vi "LoadingWindow.vi"(11 "channel":T1) -> ()   [LabVIEW 2022 SP3]
uses:
  <extravilib>/ChannelInstances/Stream-str/)Channel.ctl
  <extravilib>/ChannelInstances/Tag-bool/Read With Abort.vi
  <extravilib>/ChannelInstances/Stream-str/Read With Abort.vi
  <extravilib>/ChannelInstances/Tag-bool/Write With Abort.vi
  <extravilib>/ChannelInstances/Stream-str/EndpointRead.vi
  <extravilib>/ChannelInstances/Tag-bool/Instantiate.vi
  <extravilib>/ChannelInstances/Tag-bool/EndpointRead.vi
  <extravilib>/ChannelInstances/Stream-str/)Channel.vi
  <resource>/ChannelSupport/_ChannelSupport/WaitIfNeeded.vi
  <extravilib>/ChannelInstances/Tag-bool/Endpoint.vi
  <extravilib>/ChannelInstances/Tag-bool.lvlib
  <extravilib>/ChannelInstances/Stream-str.lvlib
panel:
  out "DescriptionBuffer":string
  out "Progress":dbl(slide) scale=0.0..14.0
  out "Description":string
  out "Task":string
  out "Version":string
  # "Ice Nucleation Controller"
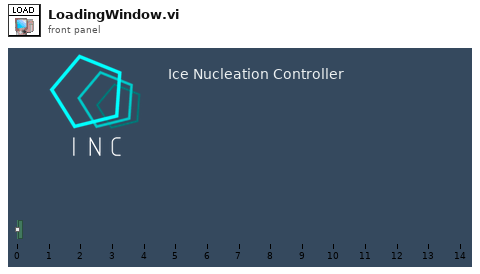
[diagram p1: front panel]
types:
  T1 = typedef "Stream-str.lvlib/)Channel.ctl" = refnum<queue>
  T2 = enum32{"Invalid", "Standard", "Closed", "Hidden", "Minimized", "Maximized"}
  T3 = enum32{"invalid app kind", "Development System", "Run Time System", "Student Edition", "Embedded LabVIEW", "Evaluation", "Custom"}
  T4 = cluster{"Core":cluster{"Current VI Reference":refnum<vi>, "Close Panel on Exit?":bool}, "Your Boolean data":bool, "Your string data":string}
  T5 = cluster{"Current VI Reference":refnum<vi>, "Close Panel on Exit?":bool}
  T6 = typedef "Tag-bool.lvlib/))Channel.ctl" = refnum<queue>
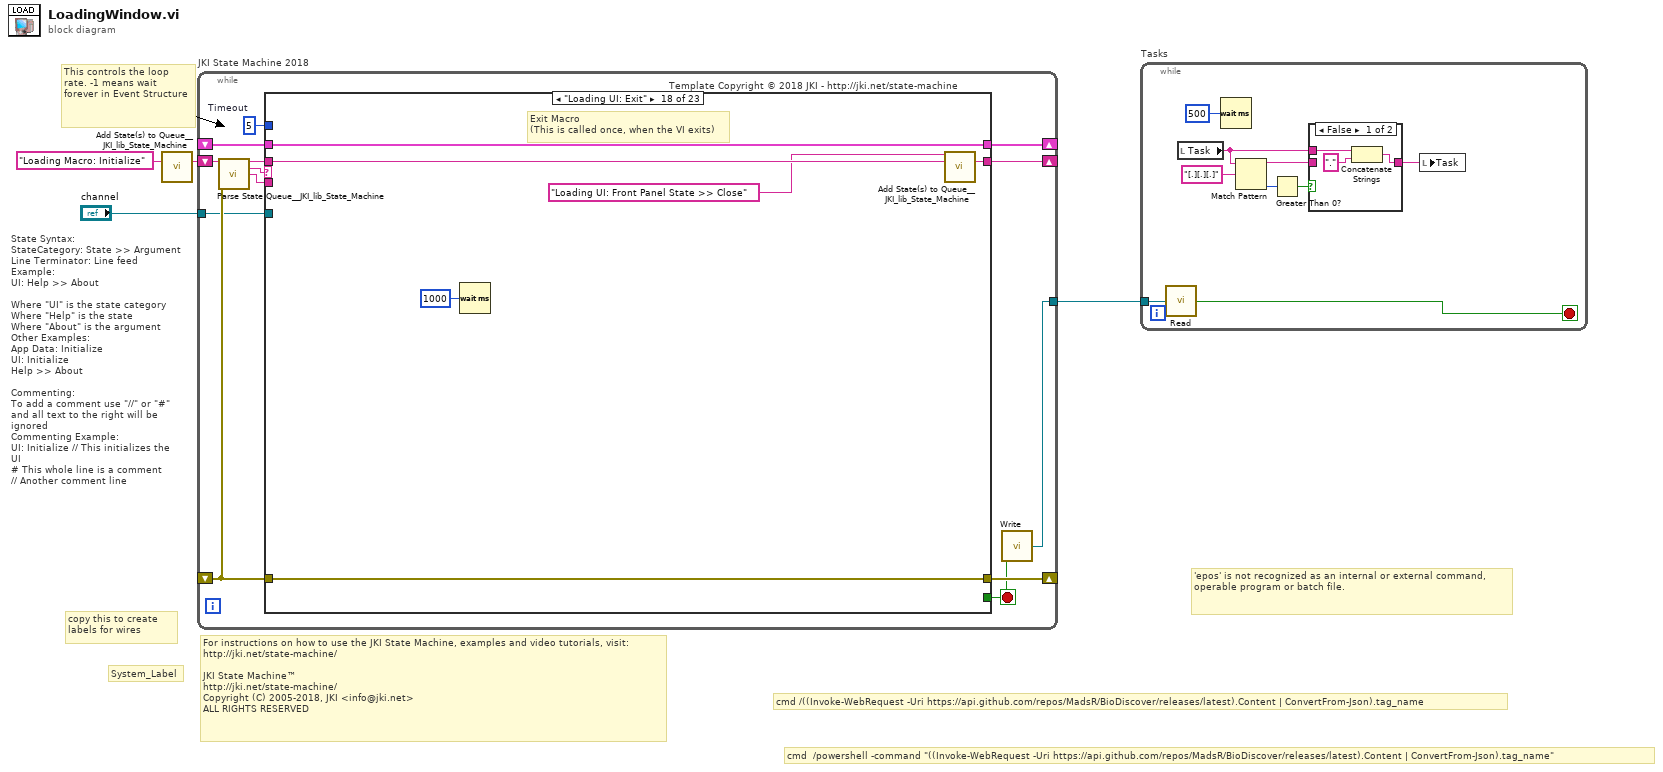
[diagram p0: block diagram]
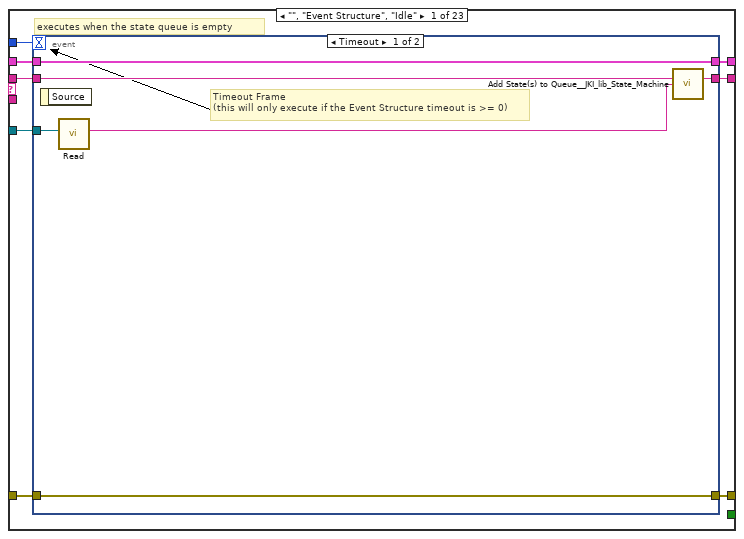
[diagram p3: hidden frame]
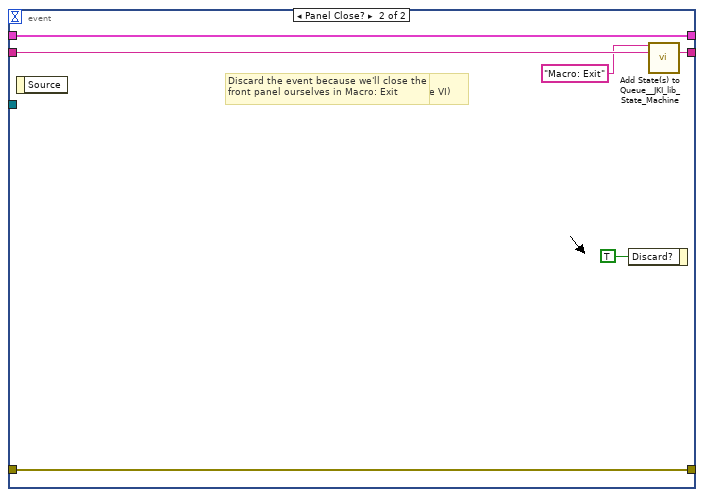
[diagram p4: hidden frame]
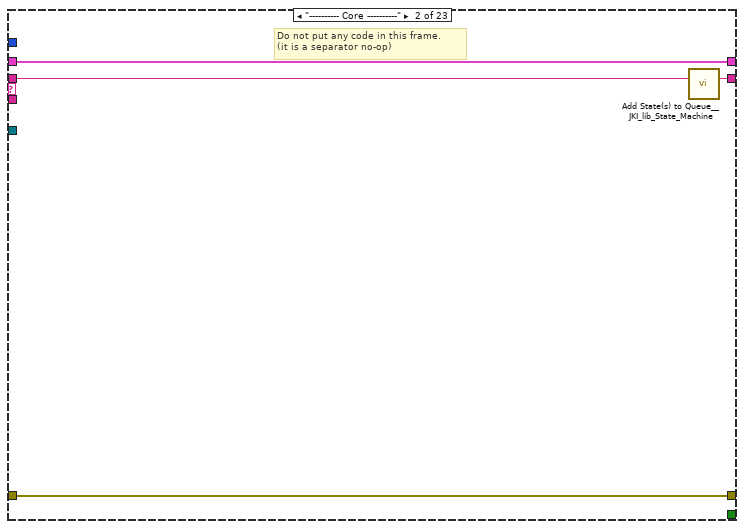
[diagram p5: hidden frame]
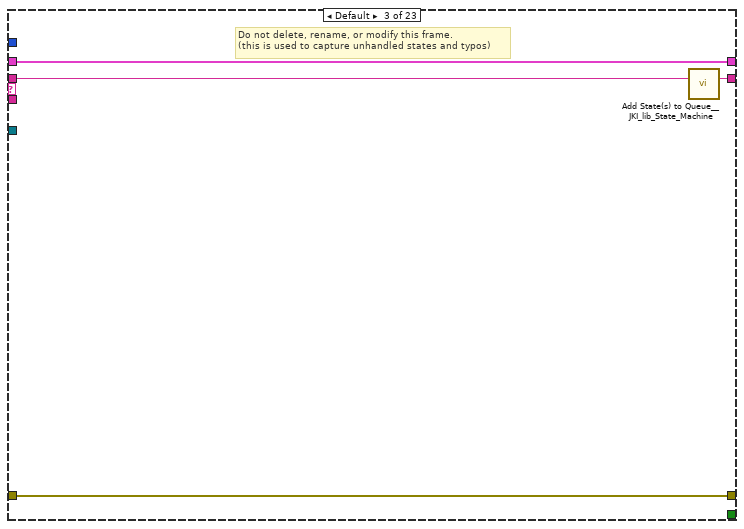
[diagram p6: hidden frame]
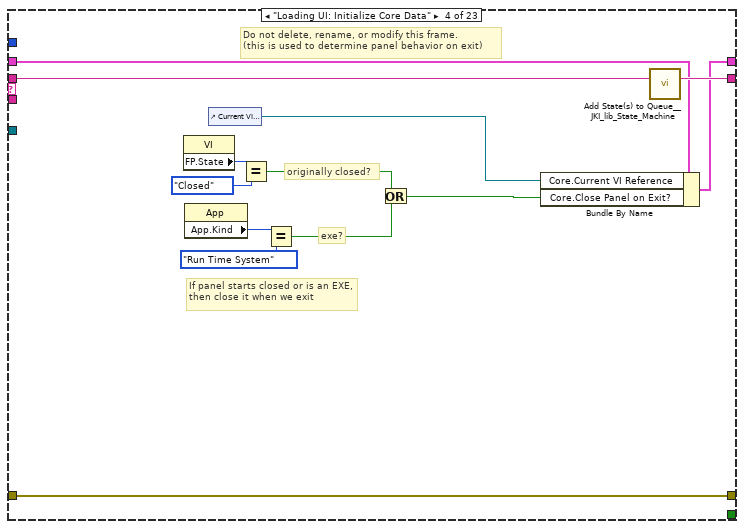
[diagram p7: hidden frame]
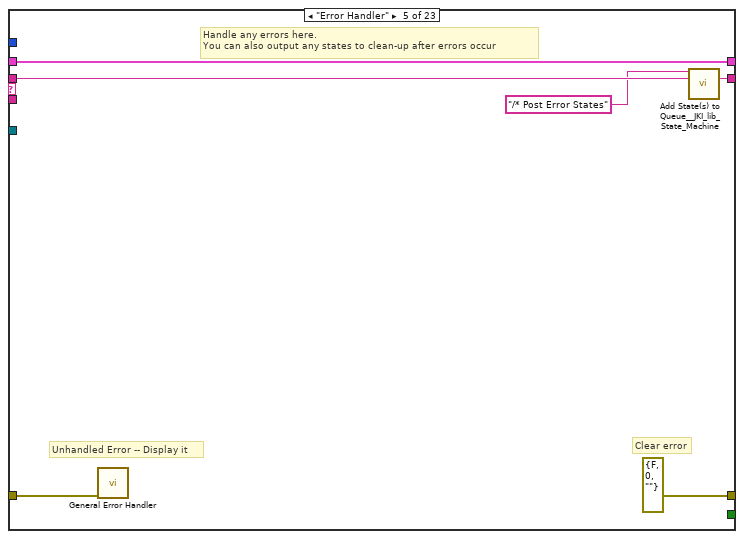
[diagram p8: hidden frame]
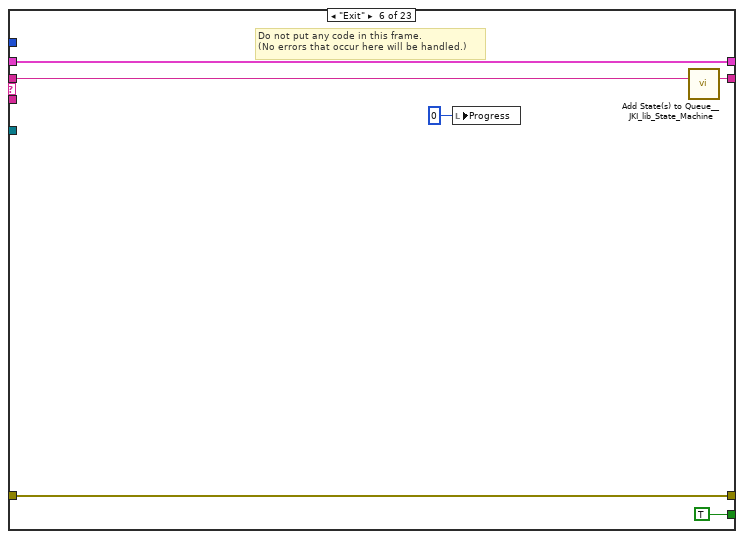
[diagram p9: hidden frame]
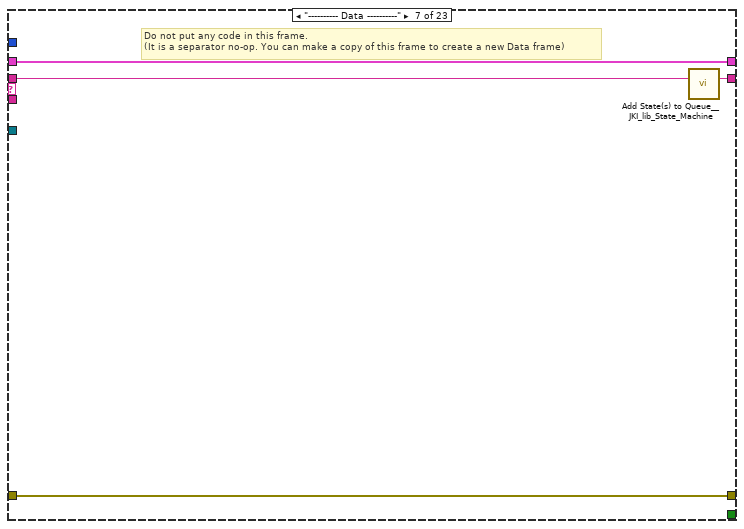
[diagram p10: hidden frame]
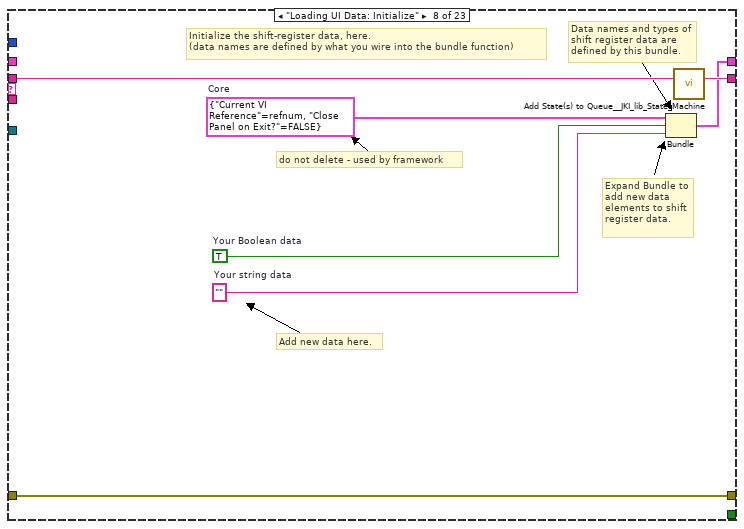
[diagram p11: hidden frame]
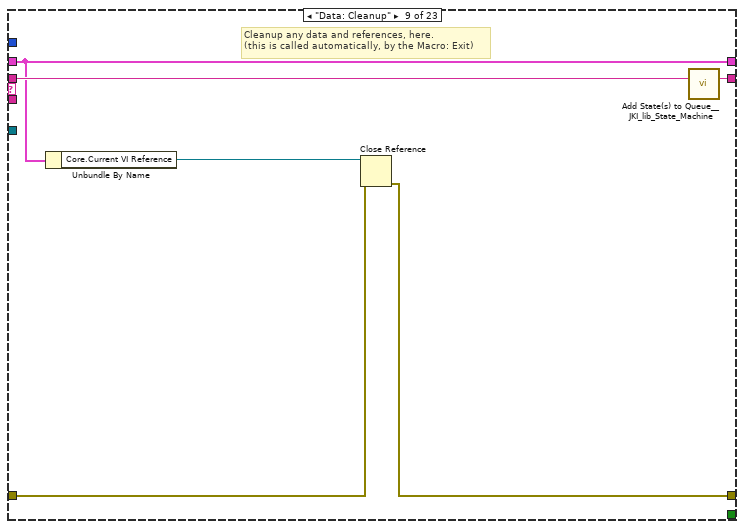
[diagram p12: hidden frame]
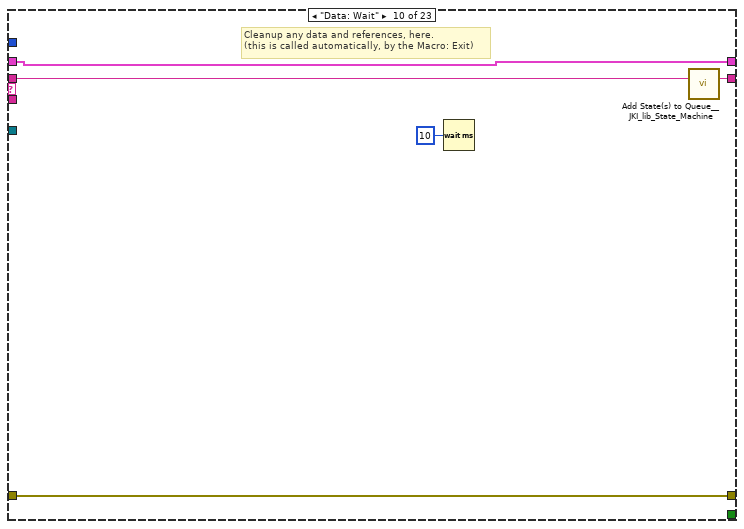
[diagram p13: hidden frame]
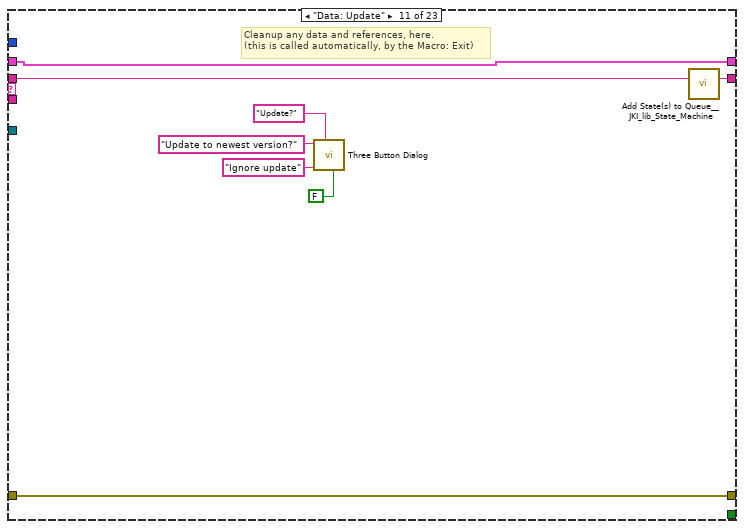
[diagram p14: hidden frame]
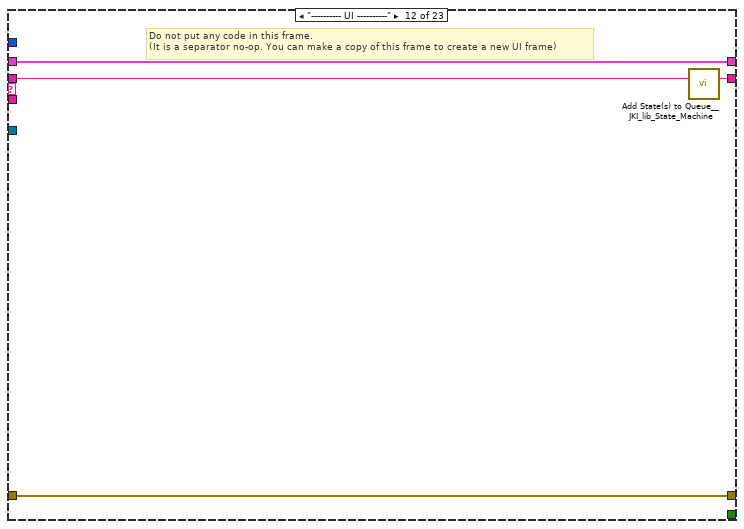
[diagram p15: hidden frame]
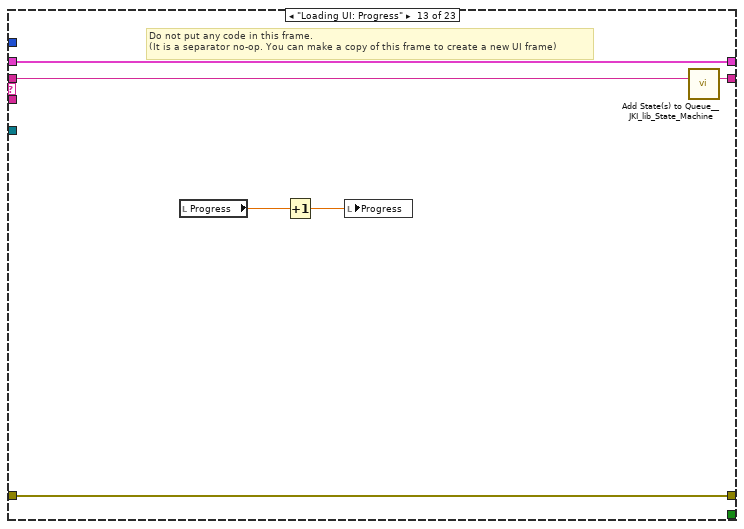
[diagram p16: hidden frame]
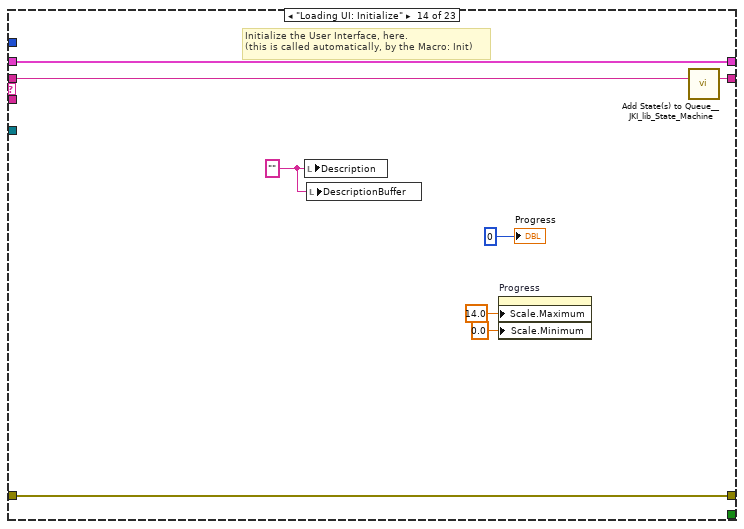
[diagram p17: hidden frame]
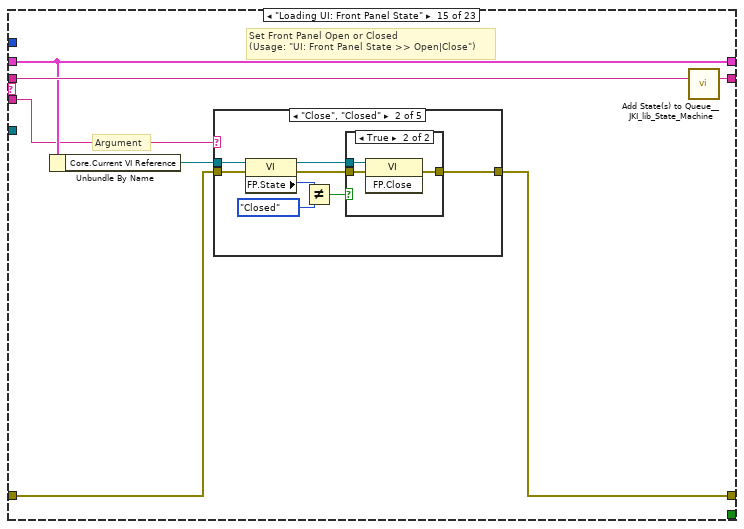
[diagram p18: hidden frame]
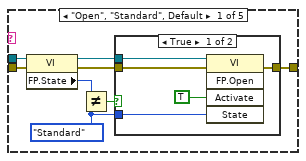
[diagram p19: hidden frame]
diagram:
  # "cmd  /powershell -command \"((Invoke-WebRequest -Uri https://api.github.com/repos/MadsR/BioDiscover/releases/latest).Content | ConvertFrom-Json).tag_name\""
  # "cmd /((Invoke-WebRequest -Uri https://api.github.com/repos/MadsR/BioDiscover/releases/latest).Content | ConvertFrom-Json).tag_name"
  # "'epos' is not recognized as an internal or external command,\noperable program or batch file."
  # "For instructions on how to use the JKI State Machine, examples and video tutorials, visit:\nhttp://jki.net/state-machine/\n\nJKI State Machine™\nhttp://jki.net/state-machine/\nCopyright (C) 2005-2018, JKI <info@jki.net>\nALL RIGHTS RESERVED"
  # "State Syntax:\nStateCategory: State >> Argument\nLine Terminator: Line feed\nExample:\nUI: Help >> About\n\nWhere \"UI\" is the state category\nWhere \"Help\" is the state\nWhere \"About\" is the argument\nOther Examples:\nApp Data: Initialize\nUI: Initialize\nHelp >> About\n\nCommenting:\nTo add a comment use \"//\" or \"#\" and all text to the right will be ignored\nCommenting Example:\nUI: Initialize // This initializes the UI\n# This whole line is a comment\n// Another comment line"
  # "copy this to create labels for wires"
  # "This controls the loop rate. -1 means wait forever in Event Structure"
  # "System_Label"
  n1 = call <vilib>:"Add State(s) to Queue__JKI_lib_State_Machine.vi"("State(s) in (\"\")"="Loading Macro: Initialize") -> ("States Out"=w4:string)  [unwired: 14 in]
  n2 = while "JKI State Machine 2018" {
    shift-right: [w10] -> _
    shift-left: _ -> [w9]
    shift-right: [w13] -> _
    shift-left: _ -> [w7]
    shift-right: [w12] -> _
    shift-left: w4 -> [w14]
    tunnel: [w6] -> w2
    tunnel: "channel" -> [w5]
    stop <- w11 stop-if-true
    w8 = 5  # Timeout
    # "Template Copyright © 2018 JKI - http://jki.net/state-machine"
    n3 = call <vilib>:"Parse State Queue__JKI_lib_State_Machine.vi"("State Queue"=w14, "Error In (no error)"=w7) -> ("Remaining States"=w16:string, "Current State"=w17:string, "Arguments"=w15:string)  [unwired: 11 in]
    n4 = case shown="\"Loading UI: Exit\"" w17 {
      tunnel: w16 -> [w25 w41 w45 w58 w64 w70 w74 w81 w87 w92 w100 w104 w110 w118 w125 w195 w204 w211 w217 w228 w233 w239 w244]
      tunnel: w15 -> [_ _ _ _ _ _ _ _ _ _ _ _ _ _ w119 w191 w197 _ w212 w223 _ _ _]
      tunnel: w9 -> [w23 w38 w43 w51 w61 w68 w71 _ w84 w89 w97 w101 w107 w116 w121 w192 w201 w208 w215 w225 w230 w236 w241]
      tunnel: [w22 w39 w42 w55 errorcluster {"status"=FALSE, "code"=0, "source"=""} ("error out") w67 w72 w78 w82 w90 w98 w102 w108 w115 w122 w193 w202 w209 w213 w226 w231 w237 w242] -> w13
      tunnel: w7 -> [w21 w39 w42 w55 w60 w67 w72 w78 w83 w90 w98 w102 w108 w115 w123 w193 w202 w209 w214 w226 w231 w237 w242]
      tunnel: [w24 w40 w44 w57 w63 w69 w73 w80 w86 w91 w99 w103 w109 w117 w124 w194 w203 w210 w216 w227 w232 w238 w243] -> w12
      tunnel: [_ _ _ _ _ TRUE _ _ _ _ _ _ _ _ _ _ _ _ _ _ _ _ _] -> w11
      tunnel: [w20 w38 w43 w56 w61 w68 w71 w79 w84 w89 w97 w101 w107 w116 w121 w192 w201 w208 w215 w225 w230 w236 w241] -> w10
      tunnel: w8 -> [w19 _ _ _ _ _ _ _ _ _ _ _ _ _ _ _ _ _ _ _ _ _ _]
      tunnel: w5 -> [w18 _ _ _ _ _ _ _ _ _ _ _ _ _ _ _ _ _ _ _ _ _ _]
      frame "", "Event Structure", "Idle" {
        # "executes when the state queue is empty"
        n5 = event shown="[0] Timeout" {
          selector: _ -> [_ _]
          dyn-events: _ -> [_ _]
          timeout: w19 -> [_ _]
          tunnel: w25 -> [w31 w37]
          tunnel: [w30 w36] -> w24
          tunnel: w23 -> [w28 w34]
          tunnel: [w29 w35] -> w22
          tunnel: w21 -> [w29 w35]
          tunnel: [w28 w34] -> w20
          tunnel: w18 -> [w27 _]
          event Timeout {
            # "Timeout Frame\n(this will only execute if the Event Structure timeout is >= 0)"
            n6 = event-data() -> ()  [unwired: 1 in, 1 out]
            n7 = call <extravilib>:"Read.vi"("channel"=w27) -> ("element"=w26:string)  [unwired: 6 in, 4 out]
            n8 = call <vilib>:"Add State(s) to Queue__JKI_lib_State_Machine.vi"("State(s) in (\"\")"=w31, "State(s) at Back (\"\")"=w26) -> ("States Out"=w30:string)  [unwired: 13 in]
          }
          event Panel Close? {
            # "Discard the event because we'll close the front panel ourselves in Macro: Exit"
            # "Close Panel button (pressed) Event\n(this executes Macro: Exit to terminate the VI)"
            n9 = event-data() -> ()  [unwired: 1 in, 1 out]
            n10 = event-data("Discard?"=TRUE) -> ()  [unwired: 1 in, 1 out]
            n11 = call <vilib>:"Add State(s) to Queue__JKI_lib_State_Machine.vi"("State(s) in Front (\"\")"="Macro: Exit", "State(s) in (\"\")"=w37) -> ("States Out"=w36:string)  [unwired: 13 in]
          }
        }
      }
      frame "---------- Core ----------" {
        # "Do not put any code in this frame.\n(it is a separator no-op)"
        n12 = call <vilib>:"Add State(s) to Queue__JKI_lib_State_Machine.vi"("State(s) in (\"\")"=w41) -> ("States Out"=w40:string)  [unwired: 14 in]
      }
      frame Default {
        # "Do not delete, rename, or modify this frame.\n(this is used to capture unhandled states and typos)"
        n13 = call <vilib>:"Add State(s) to Queue__JKI_lib_State_Machine.vi"("State(s) in (\"\")"=w45) -> ("States Out"=w44:string)  [unwired: 14 in]
      }
      frame "Loading UI: Initialize Core Data" {
        # "Do not delete, rename, or modify this frame.\n(this is used to determine panel behavior on exit)"
        # "originally closed?"
        # "exe?"
        # "If panel starts closed or is an EXE, then close it when we exit"
        n14 = property class="VI"() -> ("FP.State"=w48:T2)  [unwired: 2 in, 2 out]
        n15 = property class="App"() -> ("App.Kind"=w54:T3)  [unwired: 2 in, 2 out]
        n16 = control-ref of="Current VI Reference"() -> (w49:refnum<vi>)
        n17 = Equal?(x=w48, y=T2."Closed" ("Front Panel Window:State")) -> (x = y?=w46:bool)
        n18 = Equal?(x=w54, y=T3."Run Time System" ("Application:Kind")) -> (x = y?=w52:bool)
        n19 = Or(x=w46, y=w52) -> (x .or. y?=w50:bool)
        n20 = Bundle By Name(cluster=w51, "Core.Current VI Reference"=w49, "Core.Close Panel on Exit?"=w50) -> (w56:T4)
        n21 = call <vilib>:"Add State(s) to Queue__JKI_lib_State_Machine.vi"("State(s) in (\"\")"=w58) -> ("States Out"=w57:string)  [unwired: 14 in]
      }
      frame "Error Handler" {
        # "Unhandled Error -- Display it"
        # "Handle any errors here.\nYou can also output any states to clean-up after errors occur"
        # "Clear error"
        n22 = call <vilib>:"General Error Handler.vi"("error in (no error)"=w60) -> ()  [unwired: 10 in, 5 out]
        n23 = call <vilib>:"Add State(s) to Queue__JKI_lib_State_Machine.vi"("State(s) in Front (\"\")"="/* Post Error States", "State(s) in (\"\")"=w64) -> ("States Out"=w63:string)  [unwired: 13 in]
      }
      frame "Exit" {
        # "Do not put any code in this frame.\n(No errors that occur here will be handled.)"
        n24 = local write "Progress"(u8 0 ("Progress")) -> ()
        n25 = call <vilib>:"Add State(s) to Queue__JKI_lib_State_Machine.vi"("State(s) in (\"\")"=w70) -> ("States Out"=w69:string)  [unwired: 14 in]
      }
      frame "---------- Data ----------" {
        # "Do not put any code in this frame.\n(It is a separator no-op. You can make a copy of this frame to create a new Data frame)"
        n26 = call <vilib>:"Add State(s) to Queue__JKI_lib_State_Machine.vi"("State(s) in (\"\")"=w74) -> ("States Out"=w73:string)  [unwired: 14 in]
      }
      frame "Loading UI Data: Initialize" {
        w75 = T5 {"Current VI Reference"=refnum, "Close Panel on Exit?"=FALSE}  # Core
        w77 = TRUE  # Your Boolean data
        w76 = ""  # Your string data
        # "do not delete - used by framework"
        # "Expand Bundle to add new data elements to shift register data."
        # "Add new data here."
        # "Data names and types of shift register data are defined by this bundle."
        # "Initialize the shift-register data, here.\n(data names are defined by what you wire into the bundle function)"
        n27 = Bundle("Core"=w75, "Your Boolean data"=w77, "Your string data"=w76) -> (w79:T4)  [unwired: 1 in]
        n28 = call <vilib>:"Add State(s) to Queue__JKI_lib_State_Machine.vi"("State(s) in (\"\")"=w81) -> ("States Out"=w80:string)  [unwired: 14 in]
      }
      frame "Data: Cleanup" {
        # "Cleanup any data and references, here.\n(this is called automatically, by the Macro: Exit)"
        n29 = Unbundle By Name(w84) -> ("Core.Current VI Reference"=w85:refnum<vi>)
        n30 = Close Reference(reference=w85, error in (no error)=w83) -> (error out=w82:errorcluster)
        n31 = call <vilib>:"Add State(s) to Queue__JKI_lib_State_Machine.vi"("State(s) in (\"\")"=w87) -> ("States Out"=w86:string)  [unwired: 14 in]
      }
      frame "Data: Wait" {
        # "Cleanup any data and references, here.\n(this is called automatically, by the Macro: Exit)"
        n32 = Wait (ms)(milliseconds to wait=u32 10) -> ()  [unwired: 1 out]
        n33 = call <vilib>:"Add State(s) to Queue__JKI_lib_State_Machine.vi"("State(s) in (\"\")"=w92) -> ("States Out"=w91:string)  [unwired: 14 in]
      }
      frame "Data: Update" {
        # "Cleanup any data and references, here.\n(this is called automatically, by the Macro: Exit)"
        n34 = call <vilib>:"Three Button Dialog.vi"("Allow user to close window? (TRUE)"=FALSE, "Window Title (\"\")"="Update?" ("Window Title (\"\")"), "Right Button Text (\"Cancel\")"="Ignore update" ("Right Button Text (\"Cancel\")"), "message"="Update to newest version?") -> ()  [unwired: 7 in, 1 out]
        n35 = call <vilib>:"Add State(s) to Queue__JKI_lib_State_Machine.vi"("State(s) in (\"\")"=w100) -> ("States Out"=w99:string)  [unwired: 14 in]
      }
      frame "---------- UI ----------" {
        # "Do not put any code in this frame.\n(It is a separator no-op. You can make a copy of this frame to create a new UI frame)"
        n36 = call <vilib>:"Add State(s) to Queue__JKI_lib_State_Machine.vi"("State(s) in (\"\")"=w104) -> ("States Out"=w103:string)  [unwired: 14 in]
      }
      frame "Loading UI: Progress" {
        # "Do not put any code in this frame.\n(It is a separator no-op. You can make a copy of this frame to create a new UI frame)"
        n37 = local read "Progress"() -> (w106:dbl)
        n38 = Increment(x=w106) -> (x+1=w105:dbl)
        n39 = local write "Progress"(w105) -> ()
        n40 = call <vilib>:"Add State(s) to Queue__JKI_lib_State_Machine.vi"("State(s) in (\"\")"=w110) -> ("States Out"=w109:string)  [unwired: 14 in]
      }
      frame "Loading UI: Initialize" {
        w111 = "" ("Description")
        # "Initialize the User Interface, here.\n(this is called automatically, by the Macro: Init)"
        n41 = local write "Description"(w111) -> ()
        n42 = local write "DescriptionBuffer"(w111) -> ()
        n43 = property on="Progress" class="Slide (strict)"("Scale.Maximum"=14.0 ("Scale.Range:Maximum"), "Scale.Minimum"=0.0 ("Scale.Range:Minimum")) -> ()  [unwired: 2 in, 2 out]
        n44 = call <vilib>:"Add State(s) to Queue__JKI_lib_State_Machine.vi"("State(s) in (\"\")"=w118) -> ("States Out"=w117:string)  [unwired: 14 in]
        "Progress" <- u8 0 ("Progress")
      }
      frame "Loading UI: Front Panel State" {
        # "Argument"
        # "Set Front Panel Open or Closed\n(Usage: \"UI: Front Panel State >> Open|Close\")"
        n45 = Unbundle By Name(w121) -> ("Core.Current VI Reference"=w120:refnum<vi>)
        n46 = case shown="\"Close\", \"Closed\"" w119 {
          tunnel: w123 -> [w131 w146 w157 w170 w183]
          tunnel: [w133 w147 w159 w172 w185] -> w122
          tunnel: w120 -> [w132 w144 w158 w171 w184]
          frame "Open", "Standard", Default {
            w126 = T2."Standard" ("State")
            n47 = property class="VI"(reference=w132, error in=w131) -> (reference out=w129:refnum<vi>, error out=w130:errorcluster, "FP.State"=w128:T2)
            n48 = Not Equal?(x=w128, y=w126) -> (x != y?=w127:bool)
            n49 = case shown="True" w127 {
              tunnel: [w137 w139] -> w133
              tunnel: w130 -> [w136 w139]
              tunnel: w129 -> [w135 _]
              tunnel: w126 -> [w134 _]
              frame True {
                n50 = invoke class="VI" method="FP.Open"(reference=w135, error in=w136, "Activate"=TRUE, "State"=w134) -> (error out=w137:errorcluster)  [unwired: 1 in, 4 out]
              }
              frame False {
              }
            }
          }
          frame "Close", "Closed" {
            n51 = property class="VI"(reference=w144, error in=w146) -> (reference out=w143:refnum<vi>, error out=w145:errorcluster, "FP.State"=w141:T2)
            n52 = Not Equal?(x=w141, y=T2."Closed" ("Front Panel Window:State")) -> (x != y?=w140:bool)
            n53 = case shown="True" w140 {
              tunnel: [w148 w151] -> w147
              tunnel: w145 -> [w148 w150]
              tunnel: w143 -> [_ w149]
              frame False {
              }
              frame True {
                n54 = invoke class="VI" method="FP.Close"(reference=w149, error in=w150) -> (error out=w151:errorcluster)  [unwired: 1 in, 2 out]
              }
            }
          }
          frame "Hidden", "Hide" {
            w152 = T2."Hidden" ("State")
            n55 = property class="VI"(reference=w158, error in=w157) -> (reference out=w155:refnum<vi>, error out=w156:errorcluster, "FP.State"=w154:T2)
            n56 = Not Equal?(x=w154, y=w152) -> (x != y?=w153:bool)
            n57 = case shown="True" w153 {
              tunnel: [w163 w164] -> w159
              tunnel: w156 -> [w162 w164]
              tunnel: w155 -> [w161 _]
              tunnel: w152 -> [w160 _]
              frame True {
                n58 = invoke class="VI" method="FP.Open"(reference=w161, error in=w162, "State"=w160) -> (error out=w163:errorcluster)  [unwired: 2 in, 4 out]
              }
              frame False {
              }
            }
          }
          frame "Minimize", "Minimized" {
            w165 = T2."Minimized" ("State")
            n59 = property class="VI"(reference=w171, error in=w170) -> (reference out=w168:refnum<vi>, error out=w169:errorcluster, "FP.State"=w167:T2)
            n60 = Not Equal?(x=w167, y=w165) -> (x != y?=w166:bool)
            n61 = case shown="False" w166 {
              tunnel: [w176 w177] -> w172
              tunnel: w169 -> [w175 w177]
              tunnel: w168 -> [w174 _]
              tunnel: w165 -> [w173 _]
              frame True {
                n62 = invoke class="VI" method="FP.Open"(reference=w174, error in=w175, "State"=w173) -> (error out=w176:errorcluster)  [unwired: 2 in, 4 out]
              }
              frame False {
              }
            }
          }
          frame "Maximize", "Maximized" {
            w178 = T2."Maximized" ("State")
            n63 = property class="VI"(reference=w184, error in=w183) -> (reference out=w181:refnum<vi>, error out=w182:errorcluster, "FP.State"=w180:T2)
            n64 = Not Equal?(x=w180, y=w178) -> (x != y?=w179:bool)
            n65 = case shown="True" w179 {
              tunnel: [w189 w190] -> w185
              tunnel: w182 -> [w188 w190]
              tunnel: w181 -> [w187 _]
              tunnel: w178 -> [w186 _]
              frame True {
                n66 = invoke class="VI" method="FP.Open"(reference=w187, error in=w188, "State"=w186) -> (error out=w189:errorcluster)  [unwired: 2 in, 4 out]
              }
              frame False {
              }
            }
          }
        }
        n67 = call <vilib>:"Add State(s) to Queue__JKI_lib_State_Machine.vi"("State(s) in (\"\")"=w125) -> ("States Out"=w124:string)  [unwired: 14 in]
      }
      frame "Loading UI: Version" {
        # "Your code here.\n(You can make a copy of, or modify, this frame)"
        n68 = call <vilib>:"Add State(s) to Queue__JKI_lib_State_Machine.vi"("State(s) in (\"\")"=w195) -> ("States Out"=w194:string)  [unwired: 14 in]
        "Version" <- w191
      }
      frame "Loading UI: Description" {
        # "Your code here.\n(You can make a copy of, or modify, this frame)"
        n69 = local read "DescriptionBuffer"() -> (w196:string)
        n70 = case shown="\"Connections Successful\"" w197 {
          frame "False", Default {
          }
          frame "Connections Successful" {
            n71 = property on="Description" class="Str"("Text.TextColor"=u32 16448250 ("Text.Text Colors:Text Color")) -> ()  [unwired: 2 in, 2 out]
          }
        }
        n72 = Concatenate Strings(w196, w197) -> (w200:string)
        "Description" <- w200
        n73 = Concatenate Strings(w200, "\r\n") -> (→"DescriptionBuffer":string)
        n74 = call <vilib>:"Add State(s) to Queue__JKI_lib_State_Machine.vi"("State(s) in (\"\")"=w204) -> ("States Out"=w203:string)  [unwired: 14 in]
      }
      frame "Loading UI: Exit" {
        # "Exit Macro\n(This is called once, when the VI exits)"
        n75 = Wait (ms)(milliseconds to wait=u32 1000) -> ()  [unwired: 1 out]
        n76 = call <vilib>:"Add State(s) to Queue__JKI_lib_State_Machine.vi"("State(s) in Front (\"\")"="Loading UI: Front Panel State >> Close", "State(s) in (\"\")"=w211) -> ("States Out"=w210:string)  [unwired: 13 in]
      }
      frame "UI: Cursor Set" {
        # "Argument"
        # "Set and Unset Cursor Busy.\n(Usage: \"UI: Cursor Set >> Busy|Idle\")"
        n77 = case shown="\"Idle\", Default" w212 {
          tunnel: w214 -> [w219 w221]
          tunnel: [w218 w220] -> w213
          frame "Idle", Default {
            n78 = call <vilib>:"Unset Busy.vi"("error in (no error)"=w219) -> ("error out"=w218:errorcluster)  [unwired: 10 in]
          }
          frame "Busy" {
            n79 = call <vilib>:"Set Busy.vi"("error in (no error)"=w221) -> ("error out"=w220:errorcluster)  [unwired: 9 in, 1 out]
          }
        }
        n80 = call <vilib>:"Add State(s) to Queue__JKI_lib_State_Machine.vi"("State(s) in (\"\")"=w217) -> ("States Out"=w216:string)  [unwired: 14 in]
      }
      frame "UI: StatusString" {
        # "Your code here.\n(You can make a copy of, or modify, this frame)"
        n81 = Not Equal?(x=w223, y="Idle") -> (x != y?=w222:bool)
        n82 = case shown="True" w222 {
          tunnel: w223 -> [_ w229]
          frame False {
          }
          frame True {
            "Task" <- w229
          }
        }
        n83 = call <vilib>:"Add State(s) to Queue__JKI_lib_State_Machine.vi"("State(s) in (\"\")"=w228) -> ("States Out"=w227:string)  [unwired: 14 in]
      }
      frame "---------- Macro ----------" {
        # "Do not put any code in this frame.\n(It is a separator no-op. You can make a copy of this frame to create a new Macro frame)"
        n84 = call <vilib>:"Add State(s) to Queue__JKI_lib_State_Machine.vi"("State(s) in (\"\")"=w233) -> ("States Out"=w232:string)  [unwired: 14 in]
      }
      frame "Loading Macro: Initialize" {
        # "Initialization Macro\n(This is called once, when the VI starts)"
        n85 = property on="Description" class="Str"("Text.TextColor"=u32 16711680 ("Text.Text Colors:Text Color")) -> ()  [unwired: 2 in, 2 out]
        n86 = call <vilib>:"Add State(s) to Queue__JKI_lib_State_Machine.vi"("State(s) in Front (\"\")"="Loading UI Data: Initialize\nLoading UI: Initialize Core Data\nLoading UI: Initialize\nLoading UI: Front Panel State >> Open", "State(s) in (\"\")"=w239) -> ("States Out"=w238:string)  [unwired: 13 in]
      }
      frame "Macro: Exit" {
        # "Exit Macro\n(This is called once, when the VI exits)"
        n87 = call <vilib>:"Add State(s) to Queue__JKI_lib_State_Machine.vi"("State(s) in Front (\"\")"="Data: Cleanup\nExit", "State(s) in (\"\")"=w244) -> ("States Out"=w243:string)  [unwired: 13 in]
      }
    }
    n88 = call <extravilib>:"Write.vi"("element"=w11) -> ("channel"=w6:T6)  [unwired: 1 out]
  }
  n89 = while "Tasks" {
    tunnel: w2 -> [w253]
    stop <- w252 stop-if-true
    n90 = call <extravilib>:"Read.vi"("channel"=w253) -> ("element"=w252:bool)  [unwired: 1 in, 1 out]
    n91 = local read "Task"() -> (w247:string)
    n92 = Wait (ms)(milliseconds to wait=u32 500) -> ()  [unwired: 1 out]
    n93 = Match Pattern(string=w247, regular expression="[.][.][.]") -> (before substring=w249:string, offset past match=w248:i32)  [unwired: 1 in, 2 out]
    n94 = Greater Than 0?(x=w248) -> (x > 0?=w245:bool)
    n95 = case shown="False" w245 {
      tunnel: [w256 w257] -> w246
      tunnel: w247 -> [w254 _]
      tunnel: w249 -> [_ w257]
      frame False {
        n96 = Concatenate Strings(w254, "." ("string")) -> (w256:string)
      }
      frame True {
      }
    }
    n97 = local write "Task"(w246) -> ()
  }
